vi "Write Codes.vi"(8 "error in (no error)":errorcluster, 10 "Codes":i32[](array[numeric]), 11 "System Log in":refnum<class "System Log.lvclass">) -> (0 "error out":errorcluster, 3 "System Log out":refnum<class "System Log.lvclass">)   [LabVIEW 2016, in "System Log.lvclass"]
uses:
  System Log.lvclass
  System Log.lvclass/System Log.ctl
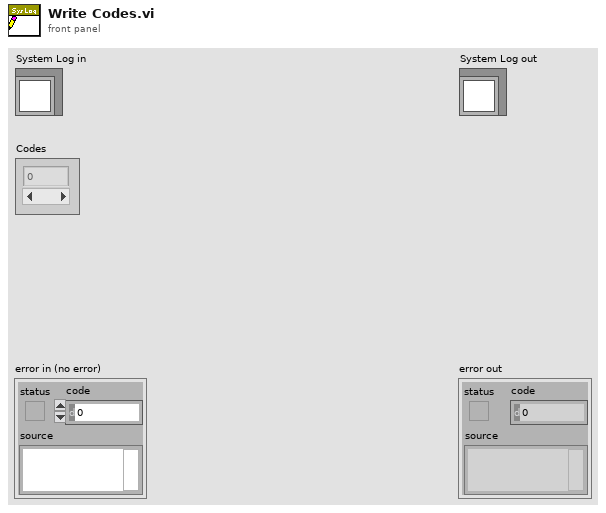
[diagram p1: front panel]
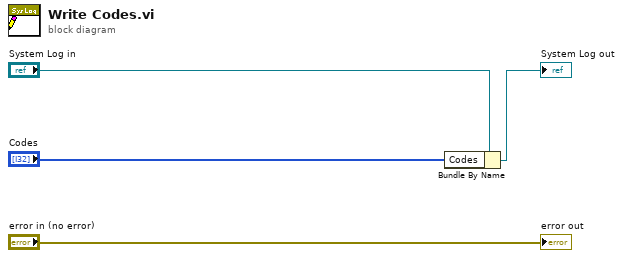
[diagram p0: block diagram]
diagram:
  n1 = Bundle By Name(cluster="System Log in", "Codes"="Codes") -> (→"System Log out":refnum<class "System Log.lvclass">)
  "error out" <- "error in (no error)"
